vi "Transfer.Total Channel Count.vi"(8 "error in (no error)":errorcluster, 10 "previous total channel count (0)":u64, 11 "Transfer in":refnum<class "Transfer.lvclass">) -> (0 "error out":errorcluster, 2 "total channel count":u64, 3 "Transfer out":refnum<class "Transfer.lvclass">)   [LabVIEW 2017, in "DSF Core.lvlib" / "Transfer.lvclass"]
uses:
  Transfer.lvclass
  Transfer.lvclass/Transfer.ctl
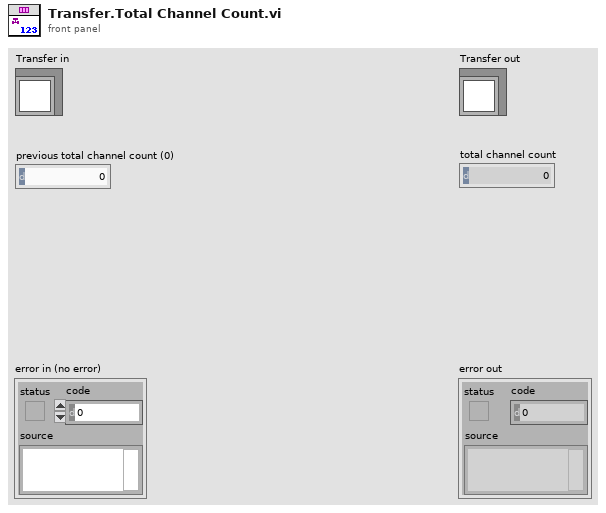
[diagram p1: front panel]
types:
  T1 = typedef "DSF Core.lvlib/DSF Runtime Channel Block.ctl" = cluster{"data type":T2, "count":u64, "buffer offset":u64}
  T2 = typedef "DSF Core.lvlib/DSF Data Type.ctl" = enum8{"Bool", "SGL", "DBL", "I8", "I16", "I32", "I64", "U8", "U16", "U32", "U64"}
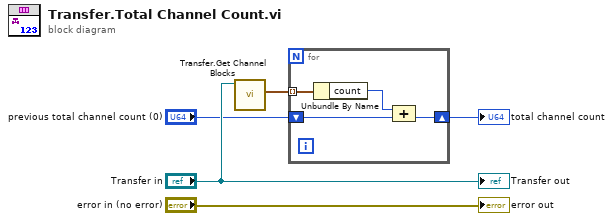
[diagram p0: block diagram]
diagram:
  n1 = call "Transfer.Get Channel Blocks.vi"("Transfer in"="Transfer in") -> ("channel blocks"=w5:T1[])  [unwired: 9 in, 1 out]
  n2 = for {
    tunnel: w5 -> [w9] mode=indexing
    shift-right: [w6] -> w2
    shift-left: "previous total channel count (0)" -> [w8]
    n3 = Unbundle By Name(w9) -> ("count"=w7:u64)
    n4 = Compound Arithmetic op=ADD(w7, w8) -> (w6:u64)
  }
  "total channel count" <- w2
  "error out" <- "error in (no error)"
  "Transfer out" <- "Transfer in"
